vi "Translation3d_Create_DistAng.vi"(10 "Angle_Quat":T1={"Q_quaternion"={"R"=1.0, "V"=[0.0, 0.0, 0.0]}}, 11 "Distance":dbl) -> (3 "TRANSLATION3D":T3 {"Z" format="%14.3f"; "Y" format="%14.3f"; "X" format="%14.3f"})   [LabVIEW 2019, in "Trajectory_Library.lvlib"]
doc: "Constructs a Translation2d with the provided distance and angle. This is essentially converting from polar coordinates to Cartesian coordinates.\n\nRepresents a translation in 2d space. This object can be used to represent a point or a vector.\n\nThis assumes that you are using conventional mathematical axes. When the robot is placed on the origin, facing toward the X direction, moving forward increases the X, whereas moving to the left increases the Y.\n\nParameters:\n - Dist - Distance.\n - Ang - Rotation representing the angle.\n\nReturns\n - TRANSLATION - The TRANSLATION data structure"
uses:
  Trajectory_Library.lvlib
  TRANSLATION3D.ctl
  ROTATION3D.ctl
  QUATERNION.ctl
  Rotation3d_GetQuaterion.vi
  Quaternion_New.vi
  Quaternion_Times.vi
  Quaternion_Inverse.vi
  Quaternion_GetLAll.vi
  Quaternion_GetLVQuat.vi
  Quaternion_New_LVQuat.vi
  Quaternion_Equals.vi
  <vilib>/robotics/Kinematics/Multiply Quaternions.vi
  <vilib>/robotics/Kinematics/Multiply Quaternion by Quaternion.vi
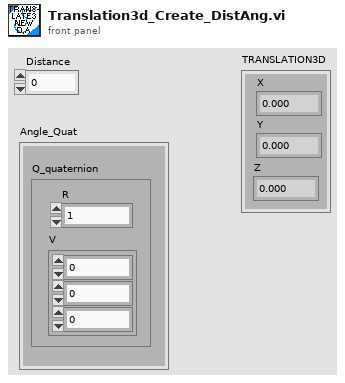
[diagram p1: front panel]
types:
  T1 = typedef "Trajectory_Library.lvlib/ROTATION3D.ctl" = cluster{"Q_quaternion":T2}
  T2 = typedef "Trajectory_Library.lvlib/QUATERNION.ctl" = cluster{"R":dbl, "V":dbl[]}
  T3 = typedef "Trajectory_Library.lvlib/TRANSLATION3D.ctl" = cluster{"X":dbl, "Y":dbl, "Z":dbl}
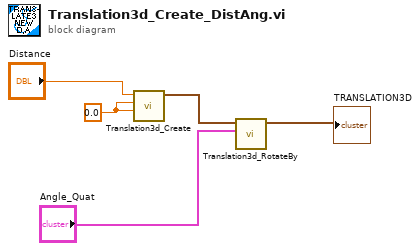
[diagram p0: block diagram]
diagram:
  w4 = 0.0 ("Y")
  n1 = call "Translation3d_Create.vi"("Z"=w4, "Y"=w4, "X"="Distance") -> ("TRANSLATION3D"=w3:T3)  [unwired: 8 in]
  n2 = call "Translation3d_RotateBy.vi"("other Rot3d"="Angle_Quat", "in Translation3D"=w3) -> ("out Translation3d"=→"TRANSLATION3D":T3)  [unwired: 9 in]
